vi "Lift to Angle.vi"(6 "Synchronization":enum16{"Start", "Wait"}(ring), 7 "Description":string, 8 "Command Info In":T1, 11 "Angle":dbl) -> (0 "Command Info Out":T1)   [LabVIEW 2019]
doc: "This template has a parameter to control whether it waits for the command to complete or not. This is useful for operations that have a timed duration or a sensor-based duration. \n\nBe sure to right-click and select New from Template and save with a new command name."
uses:
  <vilib>/Rock Robotics/WPI/Framework/Command Status Info.ctl
  <vilib>/Rock Robotics/WPI/Framework/Completion Status.ctl
  <vilib>/Rock Robotics/WPI/Framework/Completion Notifier.ctl
  Implementation/Turret Setpoints.ctl
  Implementation/Turret Operations.ctl
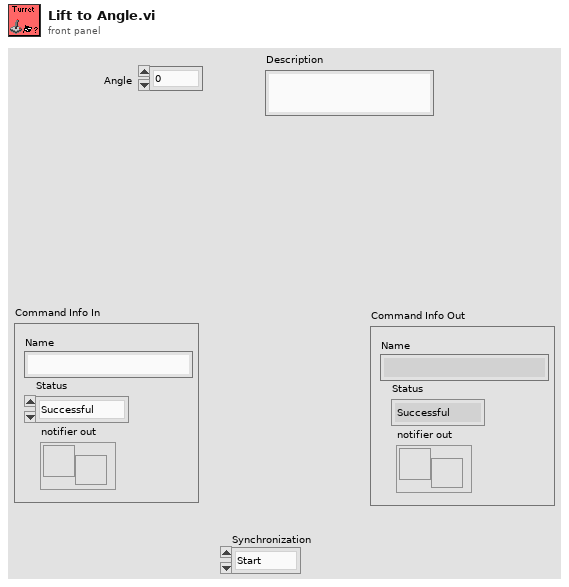
[diagram p1: front panel]
types:
  T1 = typedef "Command Status Info.ctl" = cluster{"Name":string, "Status":T2, "notifier out":T3}
  T2 = typedef "Completion Status.ctl" = enum16{"Successful", "Aborted", "Incomplete"}
  T3 = typedef "Completion Notifier.ctl" = refnum<notifier>
  T4 = typedef "Turret Setpoints.ctl" = cluster{"Operation":T5, "Angle Setpoint":dbl, "Velocity Setpoint":dbl, "Power Setpoint":dbl}
  T5 = typedef "Turret Operations.ctl" = enum16{"Reserve", "Read Current", "Immediate", "Rotate to Angle", "Align with Target", "Rotate Right Immediate", "Rotate Left Immediate", "Start Shooter", "Stop Shooter", "Lift to Angle", "Lower Immediate", "Lift Immediate"}
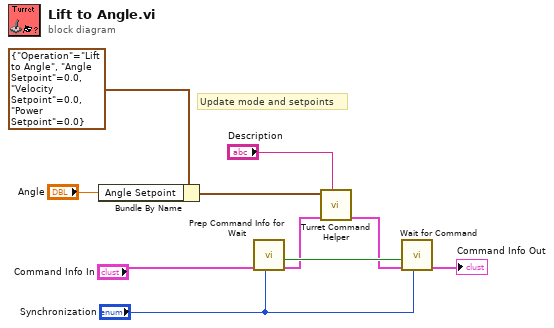
[diagram p0: block diagram]
diagram:
  # "Update mode and setpoints"
  n1 = Bundle By Name(cluster=T4 {"Operation"=enum."Lift to Angle", "Angle Setpoint"=0.0, "Velocity Setpoint"=0.0, "Power Setpoint"=0.0} ("SubSystem Data"), "Angle Setpoint"="Angle") -> (w2:T4)
  n2 = call <vilib>:"Prep Command Info for Wait.vi"("Synchronication"="Synchronization", "Command Info"="Command Info In") -> ("Command Info"=w6:T1, "Allocated"=w7:bool)  [unwired: 8 in]
  n3 = call "Turret Command Helper.vi"("Description"="Description", "Command Info In"=w6, "SubSystem Data"=w2) -> ("Command Info Out"=w3:T1)  [unwired: 6 in, 2 out]
  n4 = call <vilib>:"Wait for Command.vi"("Synchronication"="Synchronization", "Command Info in"=w3, "Allocated"=w7) -> ("Command Info out"=→"Command Info Out":T1)  [unwired: 8 in]
